vi "lqSetManifestation.vi"(8 "Error In":errorcluster, 10 "Manifestation":u64, 11 "LQIdentity in":refnum<class "LQIdentity.lvclass">) -> (0 "Error Out":errorcluster, 3 "LQIdentity out":refnum<class "LQIdentity.lvclass">)   [LabVIEW 2014, in "LQ Core.lvlib" / "LQIdentity.lvclass"]
uses:
  LQIdentity.lvclass
  LQIdentity.lvclass/LQIdentity.ctl
panel:
  # "Copyright (c) 2016 Sze Howe Koh\n\nThis Source Code Form is subject to the terms of the Mozilla Public\nLicense, v. 2.0. If a copy of the MPL was not distributed with this\nfile, You can obtain one at http://mozilla.org/MPL/2.0/."
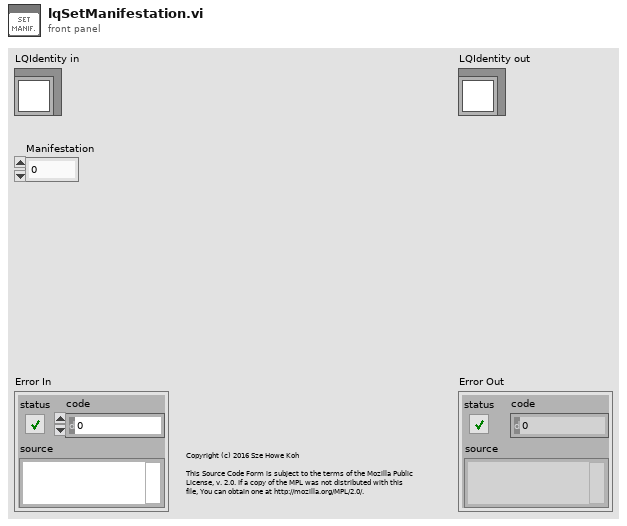
[diagram p1: front panel]
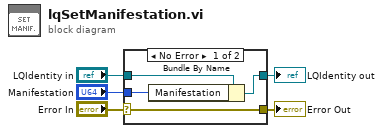
[diagram p0: block diagram]
diagram:
  n1 = case shown="No Error" "Error In" {
    selector: "Error In" -> [w6 w10]
    tunnel: "LQIdentity in" -> [w9 w11]
    tunnel: [w8 w11] -> w4
    tunnel: "Manifestation" -> [w7 _]
    tunnel: [w6 w10] -> w1
    frame No Error {
      n2 = Bundle By Name(cluster=w9, "Manifestation"=w7) -> (w8:refnum<class "LQIdentity.lvclass">)
    }
    frame Error {
    }
  }
  "LQIdentity out" <- w4
  "Error Out" <- w1
